vi "Set Fill Volume Impl.vi"(8 "error in (no error)":errorcluster, 10 "Target Volume, uL":u16, 11 "Simulated Autosampler in":refnum<class "Simulated Autosampler.lvclass">) -> (0 "error out":errorcluster, 3 "Simulated Autosampler out":refnum<class "Simulated Autosampler.lvclass">)   [LabVIEW 2023, in "Simulated Autosampler.lvlib" / "Simulated Autosampler.lvclass"]
uses:
  Simulated Autosampler.lvclass
  C:/FLASH/Development/Hardware/Autosampler/Autosampler.lvclass
  Simulated Autosampler.lvclass/Simulated Autosampler.ctl
  Autosampler/Autosampler.lvclass
  Autosampler/Autosampler State2.ctl
  Autosampler/Autosampler.lvlib
  C:/FLASH/Development/Hardware/Device/Device.lvclass
  C:/Program Files/National Instruments/LabVIEW 2023/vi.lib/ActorFramework/Actor/Actor.lvclass
  C:/FLASH/Development/Hardware/Simulated Autosampler/Simulated Autosampler.lvclass
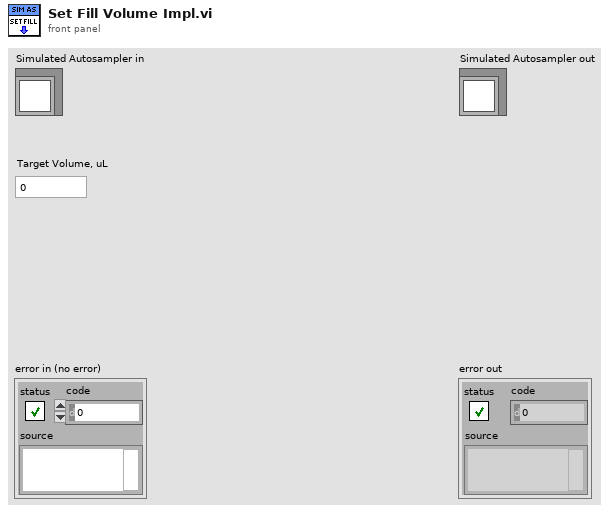
[diagram p1: front panel]
types:
  T1 = typedef "Autosampler.lvlib/Autosampler State2.ctl" = enum16{"Error", "Idle", "Positioning", "Pumping", "Shaking", "Washing", "Priming"}
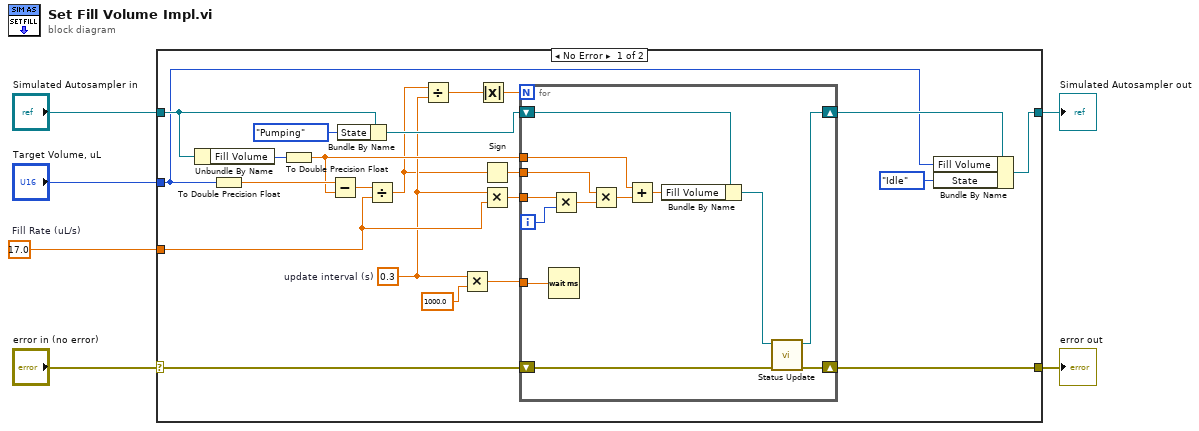
[diagram p0: block diagram]
diagram:
  w1 = 17.0  # Fill Rate (uL/s)
  n1 = case shown="No Error" "error in (no error)" {
    selector: "error in (no error)" -> [w27 w42]
    tunnel: [w26 w42] -> w5
    tunnel: "Simulated Autosampler in" -> [w21 w43]
    tunnel: [w18 w43] -> w3
    tunnel: "Target Volume, uL" -> [w17 _]
    tunnel: w1 -> [w12 _]
    frame No Error {
      w11 = 0.3  # update interval (s)
      n2 = Unbundle By Name(w21) -> ("Fill Volume"=w28:u16)
      n3 = To Double Precision Float(number=w17) -> (double precision float=w23:dbl)
      n4 = To Double Precision Float(number=w28) -> (double precision float=w14:dbl)
      n5 = Subtract(x=w23, y=w14) -> (x-y=w24:dbl)
      n6 = Bundle By Name(cluster=w21, "State"=Autosampler_State2."Pumping" ("Autosampler Status.State")) -> (w20:refnum<class "Simulated Autosampler.lvclass">)
      n7 = Divide(x=w24, y=w12) -> (x/y=w10:dbl)
      n8 = Divide(x=w10, y=w11) -> (x/y=w22:dbl)
      n9 = Multiply(x=w11, y=1000.0) -> (x*y=w16:dbl)
      n10 = Absolute Value(x=w22) -> (abs(x)=w25:dbl)
      n11 = Sign(1:w10) -> (0:w9:dbl)
      n12 = Multiply(x=w11, y=w12) -> (x*y=w13:dbl)
      n13 = for {
        N: w25 -> [_]
        shift-right: [w40] -> w26
        shift-left: w27 -> [w41]
        shift-right: [w37] -> w19
        shift-left: w20 -> [w39]
        tunnel: w16 -> [w36]
        tunnel: w13 -> [w35]
        tunnel: w14 -> [w32]
        tunnel: w9 -> [w31]
        i -> [w34]
        n14 = Wait (ms)(milliseconds to wait=w36) -> ()  [unwired: 1 out]
        n15 = Multiply(x=w35, y=w34) -> (x*y=w30:dbl)
        n16 = Multiply(x=w31, y=w30) -> (x*y=w29:dbl)
        n17 = Add(x=w32, y=w29) -> (x+y=w33:dbl)
        n18 = Bundle By Name(cluster=w39, "Fill Volume"=w33) -> (w38:refnum<class "Simulated Autosampler.lvclass">)
        n19 = call "Status Update.vi"("error in (no error)"=w41, "Autosampler in"=w38) -> ("error out"=w40:errorcluster, "Autosampler out"=w37:refnum<class "Simulated Autosampler.lvclass">)  [unwired: 7 in, 1 out]
      }
      n20 = Bundle By Name(cluster=w19, "Fill Volume"=w17, "State"=Autosampler_State2."Idle" ("Autosampler Status.State")) -> (w18:refnum<class "Simulated Autosampler.lvclass">)
    }
    frame Error {
    }
  }
  "error out" <- w5
  "Simulated Autosampler out" <- w3
